vi "Image Display And Save.vi"() -> ()   [LabVIEW 2018]
doc: "Image Display And Save: This example is an example of image reading, display, and saving. It uses attribute nodes to display images and uses the imwrite.vi function to save the images to a file."
uses:
  vi.lib/VIRobotics/opencv_yiku/ctls/ColorConversionCodes.ctl
  vi.lib/VIRobotics/opencv_yiku/Mat/Mat_8U/Mat_8U.lvclass
  D:/Program Files/company/National Instruments/LabVIEW 2018/vi.lib/addons/VIRobotics/opencv_yiku/Mat/Mat/Mat.lvclass
  vi.lib/VIRobotics/opencv_yiku/Mat/Create_Mat_8U.vi
  vi.lib/VIRobotics/opencv_yiku/Mat/Mat/Mat_release.vi
  vi.lib/VIRobotics/opencv_yiku/opencv_yiku.lvlib
  vi.lib/VIRobotics/opencv_yiku/Mat/Mat/Mat.lvclass
panel:
  out "src out":picture
  out "dst out":picture
  # "Overview: Demonstrates how to load an image, display it in a picture control, and save it to a file.\nRequirements: Windows.\nInstructions: \n1. Run the VI."
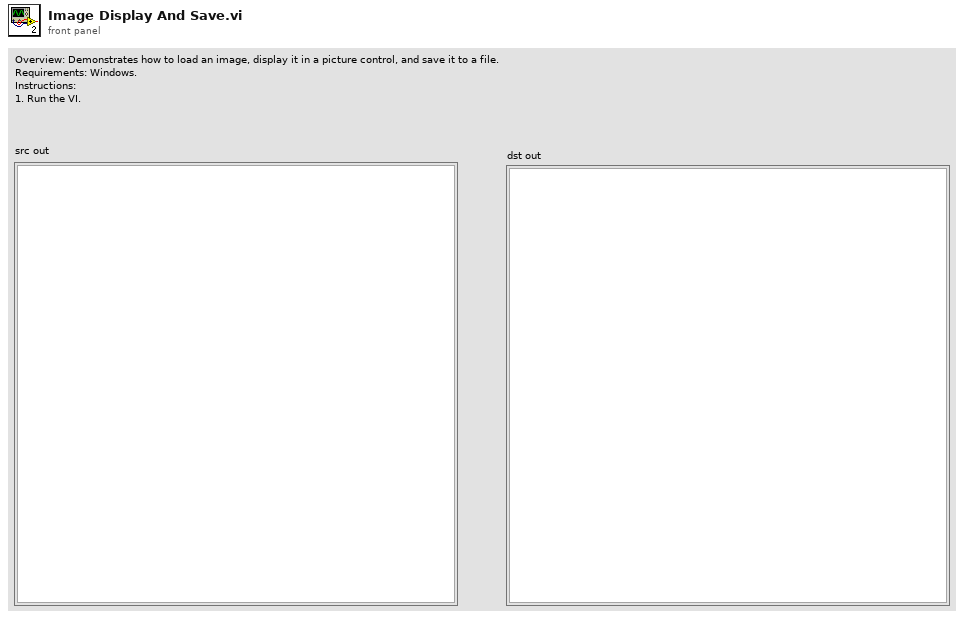
[diagram p1: front panel]
types:
  T1 = typedef "opencv_yiku.lvlib/ColorConversionCodes.ctl" = enum32{"COLOR_BGR2BGRA", "COLOR_BGRA2BGR", "COLOR_BGR2RGBA", "COLOR_RGBA2BGR", "COLOR_BGR2RGB", "COLOR_BGRA2RGBA", "COLOR_BGR2GRAY", "COLOR_RGB2GRAY", "COLOR_GRAY2BGR", "COLOR_GRAY2BGRA", "COLOR_BGRA2GRAY", "COLOR_RGBA2GRAY", "COLOR_BGR2BGR565", "COLOR_RGB2BGR565", "COLOR_BGR5652BGR", "COLOR_BGR5652RGB", "COLOR_BGRA2BGR565", "COLOR_RGBA2BGR565", "COLOR_BGR5652BGRA", "COLOR_BGR5652RGBA", "COLOR_GRAY2BGR565", "COLOR_BGR5652GRAY", "COLOR_BGR2BGR555", "COLOR_RGB2BGR555", "COLOR_BGR5552BGR", "COLOR_BGR5552RGB", "COLOR_BGRA2BGR555", "COLOR_RGBA2BGR555", "COLOR_BGR5552BGRA", "COLOR_BGR5552RGBA", "COLOR_GRAY2BGR555", "COLOR_BGR5552GRAY", "COLOR_BGR2XYZ", "COLOR_RGB2XYZ", "COLOR_XYZ2BGR", "COLOR_XYZ2RGB", "COLOR_BGR2YCrCb", "COLOR_RGB2YCrCb", "COLOR_YCrCb2BGR", "COLOR_YCrCb2RGB", "COLOR_BGR2HSV", "COLOR_RGB2HSV", "42", "43", "COLOR_BGR2Lab", "COLOR_RGB2Lab"}
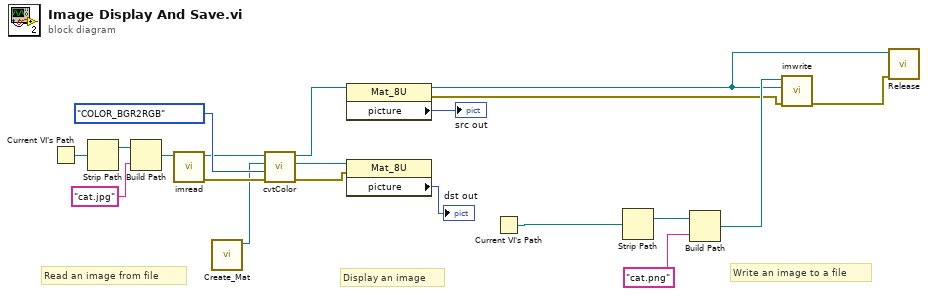
[diagram p0: block diagram]
diagram:
  # "Write an image to a file"
  # "Display an image"
  # "Read an image from file"
  n1 = Current VI's Path() -> (path=w20:path)
  n2 = Strip Path(path=w20) -> (stripped path=w19:path)  [unwired: 1 out]
  n3 = Build Path(base path=w19, name or relative path="cat.jpg") -> (appended path=w17:path)
  n4 = call "imread.vi"("path"=w17) -> ("error out"=w14:errorcluster, "Mat out"=w11:refnum<class "Mat_8U.lvclass">)  [unwired: 9 in]
  n5 = call-poly "Create_Mat.vi"() -> ("Mat_8U_out"=w8:refnum<class "Mat_8U.lvclass">)  [unwired: 10 in, 1 out]
  n6 = call "cvtColor.vi"("error in (no error)"=w14, "dstCn"=ColorConversionCodes."COLOR_BGR2RGB", "dst"=w8, "src"=w11) -> ("error out"=w13:errorcluster, "dst out"=w12:refnum<class "Mat_8U.lvclass">, "src out"=w9:refnum<class "Mat_8U.lvclass">)  [unwired: 5 in]
  n7 = property class="Mat_8U"(reference=w9) -> (reference out=w2:refnum<class "Mat_8U.lvclass">, error out=w3:errorcluster, "picture"=→"src out":picture)  [unwired: 1 in]
  n8 = property class="Mat_8U"(reference=w12, error in=w13) -> ("picture"=→"dst out":picture)  [unwired: 2 out]
  n9 = Current VI's Path() -> (path=w7:path)
  n10 = Strip Path(path=w7) -> (stripped path=w6:path)  [unwired: 1 out]
  n11 = Build Path(base path=w6, name or relative path="cat.png") -> (appended path=w4:path)
  n12 = call "imwrite.vi"("error in (no error)"=w3, "Mat out"=w2, "path"=w4) -> ("error out"=w1:errorcluster)  [unwired: 8 in]
  n13 = call-poly "Release.vi"("error in (no error)"=w1, "Mat in"=w2) -> ()  [unwired: 9 in, 1 out]
